vi "CE Do Single Measurement.vi"(6 "Iteration index":i32, 7 "TWM handle in":i32, 8 "error in (no error)":errorcluster, 9 "CE measurement":T1={"Signal frequencies (Hz) T"=[1000.0], "Signal amplitudes (V) T"=[0.707], "Sampling frequencies (Hz) T"=[10000000.0], "Record lengths (multiples of periods) T"=[10000.0], "TWM data root directory"=path "", "TWM mreasurements directories"=[], "Calculate RMS from samples"=FALSE, "Algorithm to use"="TWM-WFFT", "Quantity to read"="TWM-WFFT", "Settle down after AC source change (s) T"=1.0, "Skip PJVS setup"=FALSE, "Measurement template file"=path "", "Row of START keyword T"=0, "Row of STOP keyword T"=0, "Measurement template line T"=[], "Switch position T"=[10000.0], "FR fit mat file T"=path "", "Recalculate-skip already calculated"=FALSE} {"Switch position T" format="%#_3p"; "Record lengths (multiples of periods) T" format="%#_3p"; "Sampling frequencies (Hz) T" format="%#_3p"; "Signal amplitudes (V) T" format="%#_3p"; "Signal frequencies (Hz) T" format="%#_3p"}, 10 "Common properties":T2={"Measurement status ref"=refnum, "TWM Status ref"=refnum, "Abort ref"=refnum, "Skip waiting ref"=refnum, "GNU Octave path"=path "C:/Program Files/GNU Octave/Octave-6.2.0/mingw64/bin", "TWM+QWTB path"=path "C:/Users/labina/Desktop/TWM-1.8.7.0-full/octprog", "lvlib path"=path "D:/martin/WAC/WACsw - github/control_software/Filter function meter/external libraries/GOLPI 0.7.3.1 source distribution LV 20.0 32 bit/lv_proc.dll", "TWM pipe"="\\\\.\\pipe\\TWM:server", "PJVS status ref"=refnum, "WAC path"=path ""}) -> (0 "error out":errorcluster, 1 "TWM result as string":string[][](array[string]), 2 "TWM result as number":dbl[][](array[numeric]), 5 "TWM handle out":i32)   [LabVIEW 2020]
doc: "Setup TWM for single CE measurement, start TWM and read output."
uses:
  Utilities/Type definitions/Common properties.ctl
  Type definitions/CE measurement.ctl
  Utilities/Type definitions/Sampling properties.ctl
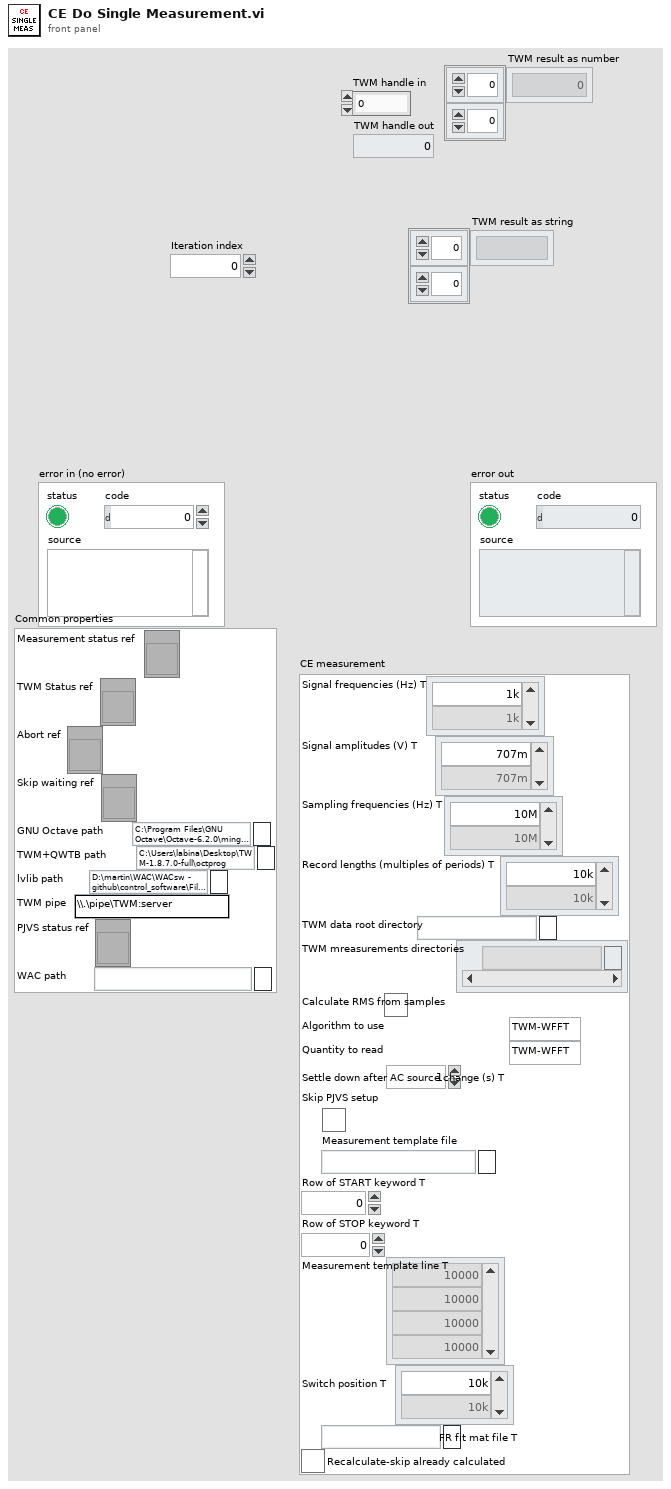
[diagram p1: front panel]
types:
  T1 = typedef "CE measurement.ctl" = cluster{"Signal frequencies (Hz) T":dbl[], "Signal amplitudes (V) T":dbl[], "Sampling frequencies (Hz) T":dbl[], "Record lengths (multiples of periods) T":dbl[], "TWM data root directory":path, "TWM mreasurements directories":path[], "Calculate RMS from samples":bool, "Algorithm to use":string, "Quantity to read":string, "Settle down after AC source change (s) T":dbl, "Skip PJVS setup":bool, "Measurement template file":path, "Row of START keyword T":i32, "Row of STOP keyword T":i32, "Measurement template line T":i32[], "Switch position T":dbl[], "FR fit mat file T":path, "Recalculate-skip already calculated":bool}
  T2 = typedef "Common properties.ctl" = cluster{"Measurement status ref":refnum<vi>, "TWM Status ref":refnum<vi>, "Abort ref":refnum<vi>, "Skip waiting ref":refnum<vi>, "GNU Octave path":path, "TWM+QWTB path":path, "lvlib path":path, "TWM pipe":string, "PJVS status ref":refnum<vi>, "WAC path":path}
  T3 = typedef "Sampling properties.ctl" = cluster{"Sampling frequency (Hz)":dbl, "Record length (multiples of period)":dbl, "Signal amplitude (V)":dbl, "Measurement frequency (Hz)":dbl, "Calculate RMS from samples":bool, "Algorithm":string, "Quantity":string, "Measurement path":string}
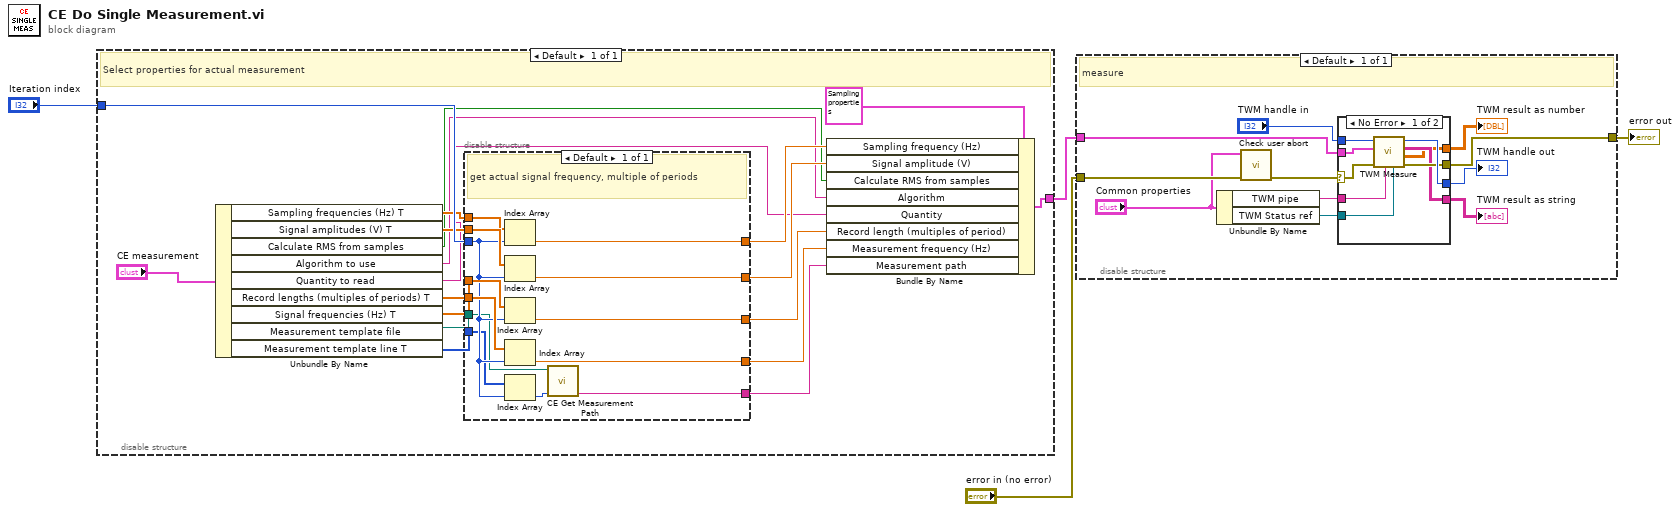
[diagram p0: block diagram]
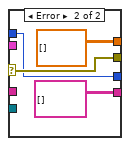
[diagram p2: hidden frame]
diagram:
  n1 = disable-structure shown="Default" {
    disable-tunnel: "Iteration index" -> [w19]
    disable-tunnel: [w20] -> w4
    frame Enabled {
      # "Select properties for actual measurement"
      n2 = Unbundle By Name("CE measurement") -> ("Sampling frequencies (Hz) T"=w15:dbl[], "Signal amplitudes (V) T"=w14:dbl[], "Calculate RMS from samples"=w13:bool, "Algorithm to use"=w12:string, "Quantity to read"=w5:string, "Record lengths (multiples of periods) T"=w11:dbl[], "Signal frequencies (Hz) T"=w10:dbl[], "Measurement template file"=w6:path, "Measurement template line T"=w7:i32[])
      n3 = disable-structure shown="Default" {
        disable-tunnel: w10 -> [w35]
        disable-tunnel: w11 -> [w34]
        disable-tunnel: w19 -> [w27]
        disable-tunnel: [w33] -> w18
        disable-tunnel: [w32] -> w22
        disable-tunnel: w14 -> [w31]
        disable-tunnel: [w30] -> w17
        disable-tunnel: w15 -> [w29]
        disable-tunnel: [w28] -> w16
        disable-tunnel: [w23] -> w9
        disable-tunnel: w7 -> [w26]
        disable-tunnel: w6 -> [w24]
        frame Enabled {
          # "get actual signal frequency, multiple of periods"
          n4 = Index Array(array=w29, index=w27) -> (element=w28:dbl)
          n5 = Index Array(array=w31, index=w27) -> (element=w30:dbl)
          n6 = Index Array(array=w34, index=w27) -> (element=w32:dbl)
          n7 = Index Array(array=w35, index=w27) -> (element=w33:dbl)
          n8 = Index Array(array=w26, index=w27) -> (element=w25:i32)
          n9 = call "CE Get Measurement Path.vi"("Template line"=w25, "Measurement template file"=w24) -> ("Measurement path as string"=w23:string)  [unwired: 8 in, 1 out]
        }
      }
      n10 = Bundle By Name(cluster=T3 {"Sampling frequency (Hz)"=500000.0, "Record length (multiples of period)"=1000.0, "Signal amplitude (V)"=4.5, "Measurement frequency (Hz)"=1000.0, "Calculate RMS from samples"=FALSE, "Algorithm"="TWM-WFFT", "Quantity"="rms", "Measurement path"=""} ("TWM Measurement properties"), "Sampling frequency (Hz)"=w16, "Signal amplitude (V)"=w17, "Calculate RMS from samples"=w13, "Algorithm"=w12, "Quantity"=w5, "Record length (multiples of period)"=w22, "Measurement frequency (Hz)"=w18, "Measurement path"=w9) -> (w20:T3)
    }
  }
  n11 = disable-structure shown="Default" {
    disable-tunnel: "error in (no error)" -> [w46]
    disable-tunnel: [w39] -> w3
    disable-tunnel: w4 -> [w45]
    frame Enabled {
      # "measure"
      n12 = Unbundle By Name("Common properties") -> ("TWM pipe"=w43:string, "TWM Status ref"=w42:refnum<vi>)
      n13 = call "Check user abort.vi"("error in (no error)"=w46, "Common properties"="Common properties") -> ("error out"=w36:errorcluster)  [unwired: 9 in]
      n14 = case shown="No Error" w36 {
        selector: w36 -> [w47 w59]
        tunnel: w45 -> [w55 _]
        tunnel: w43 -> [w54 _]
        tunnel: w42 -> [w53 _]
        tunnel: "TWM handle in" -> [w52 w57]
        tunnel: [w51 w57] -> w40
        tunnel: [w50 w59] -> w39
        tunnel: [w49 string[][] [] ("TWM result as string")] -> w38
        tunnel: [w48 dbl[][] [] ("TWM result as number")] -> w37
        frame No Error {
          n15 = call "TWM Measure.vi"("TWM Status ref"=w53, "TWM pipe"=w54, "error in (no error)"=w47, "TWM Measurement properties"=w55, "TWM handle"=w52) -> ("error out"=w50:errorcluster, "TWM result as number"=w48:dbl[][], "TWM result as string"=w49:string[][], "TWM handle out"=w51:i32)  [unwired: 3 in]
        }
        frame Error {
        }
      }
      "TWM handle out" <- w40
      "TWM result as string" <- w38
      "TWM result as number" <- w37
    }
  }
  "error out" <- w3
